vi "decision_function.vi"(8 "error in (no error)":errorcluster caption="entrée d'erreur (pas d'erreur)", 11 "RidgeClassifierCV.lvclass 2":refnum<class "RidgeClassifierCV.lvclass">) -> (0 "error out":errorcluster caption="sortie d'erreur", 2 "conf":dbl[][](array[numeric]), 3 "RidgeClassifierCV.lvclass":refnum<class "RidgeClassifierCV.lvclass">)   [LabVIEW 2020, in "RidgeClassifierCV.lvclass"]
doc: "Predict confidence scores for samples.\n\n The confidence score for a sample is proportional to the signed\n distance of that sample to the hyperplane."
uses:
  RidgeClassifierCV.lvclass
  C:/Users/cipop/TDF Dropbox/2_Technologies de France/1 - Services et Etudes/PLAIY/2 - DEV/PLAIYLAB/code/Python/Python.lvclass
  C:/Users/cipop/TDF Dropbox/2_Technologies de France/1 - Services et Etudes/PLAIY/2 - DEV/PLAIYLAB/code/Model/Model.lvclass
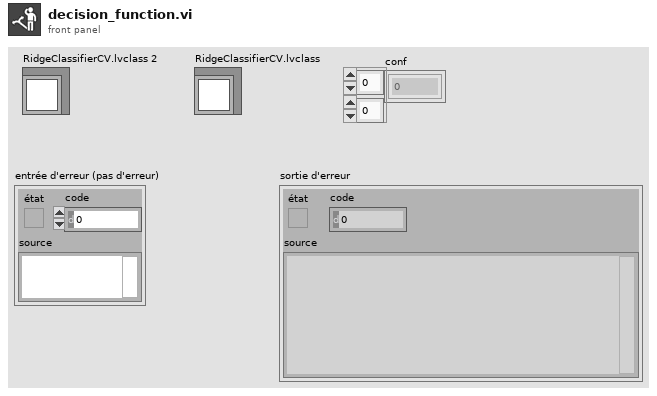
[diagram p1: front panel]
types:
  T1 = typedef "data.ctl" = cluster{"name":string, "X":dbl[][]}
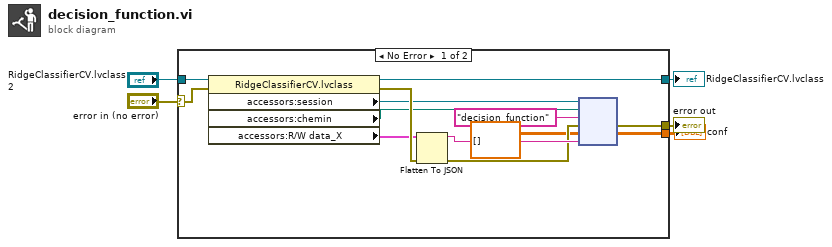
[diagram p0: block diagram]
diagram:
  n1 = case shown="No Error" "error in (no error)" {
    selector: "error in (no error)" -> [w16 w20]
    tunnel: [w17 w20] -> w4
    tunnel: [w9 w19] -> w2
    tunnel: "RidgeClassifierCV.lvclass 2" -> [w8 w19]
    tunnel: [w6 _] -> w1
    frame No Error {
      n2 = property class="RidgeClassifierCV.lvclass"(reference=w8, error in=w16) -> (reference out=w9:refnum<class "RidgeClassifierCV.lvclass">, error out=w14:errorcluster, "accessors:session"=w11:refnum<k35>, "accessors:chemin"=w10:path, "accessors:R/W data_X"=w12:T1)
      n3 = Flatten To JSON(anything=w12, error in (no error)=w14) -> (JSON string=w15:string, 11:w13:errorcluster)  [unwired: 1 in]
      n4 = node(w11, w10, "decision_function" ("nom de la fonction"), w13, dbl[][] [], w15) -> (w17:errorcluster, w6:dbl[][])  [unwired: 1 in, 3 out]
    }
    frame Error {
    }
  }
  "error out" <- w4
  "RidgeClassifierCV.lvclass" <- w2
  "conf" <- w1
